vi "IMS Stepper Set Zero.vi"(0 "Instrument Address":refnum<visa-resource-name>, 1 "Motor Number":u32=1 min=1 max=255 step=1, 2 "error in (no error)":errorcluster) -> (3 "Instrument Address Out":refnum<visa-resource-name>, 6 "error out":errorcluster)   [LabVIEW 2019]
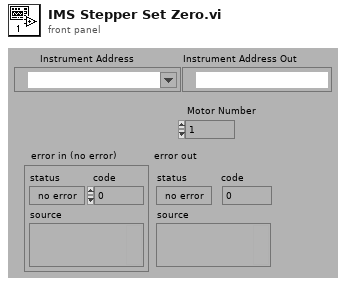
[diagram p1: front panel]
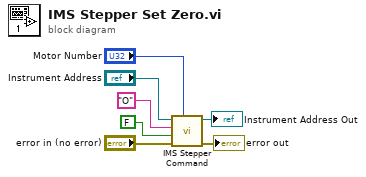
[diagram p0: block diagram]
diagram:
  n1 = call "IMS Stepper Command.vi"("Motor Number"="Motor Number", "error in (no error)"="error in (no error)", "Mode"=FALSE, "Command"="O", "Instrument Address"="Instrument Address") -> ("error out"=→"error out":errorcluster, "Instrument Address Out"=→"Instrument Address Out":refnum<visa-resource-name>)  [unwired: 1 in, 2 out]
